vi "AxisControl.vi"(0 "String in":string, 1 "AxisBounds":T5={"Min"={"Auto"=TRUE, "Value"=0.0}, "Max"={"Auto"=TRUE, "Value"=0.0}}, 2 "Time Format String":string, 3 "ticsAndGrids":T2={"tics"={"ticMin"=0.0, "ticStep"=0.0, "ticMax"=0.0, "minorDivsPerMajor"=2, "ticSpacing"=enum."Auto Tics", "ticPosition"=enum."Inside, no mirror"}, "Grids"={"Gridlines"=enum."Major grid", "Zeroaxis"=enum."No zero axis"}, "Mapping"=enum."Lin"}, 5 "Axis":T7="x", 7 "Time format?":bool, 9 "ShowNumbers?":bool=TRUE, 11 "ShowLabel?":bool=TRUE, 12 "Axis Label":string, 13 "DataSpan":cluster{"Max":dbl, "Min":dbl}, 14 "AdditionalTics":dbl[](array[numeric])) -> (4 "String out":string, 6 "Commands":T1)   [LabVIEW 2015]
uses:
  axisName.ctl
  minAndMax.ctl
  AutoManualNumber.ctl
  ticsAndGrids.ctl
  tics.ctl
  grids.ctl
  commandArray.ctl
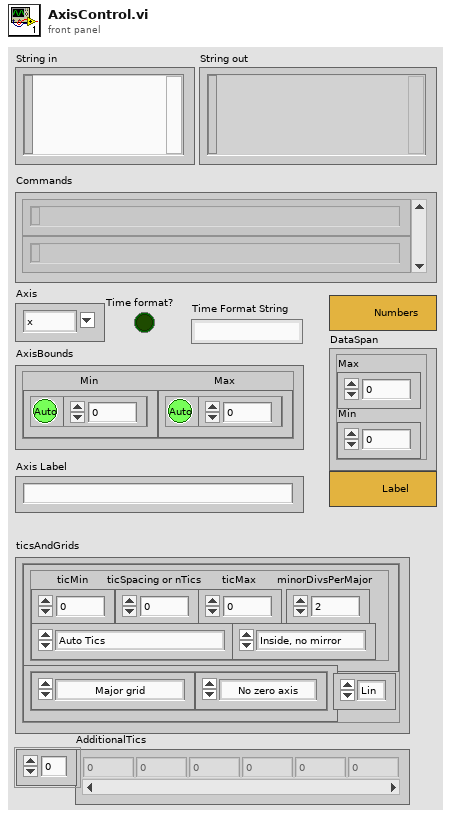
[diagram p1: front panel]
types:
  T1 = typedef "commandArray.ctl" = string[]
  T2 = typedef "ticsAndGrids.ctl" = cluster{"tics":T3, "Grids":T4, "Mapping":enum8{"Lin", "Log"}}
  T3 = typedef "tics.ctl" = cluster{"ticMin":dbl, "ticStep":dbl, "ticMax":dbl, "minorDivsPerMajor":i32, "ticSpacing":enum16{"Auto Tics", "Fixed spacing", "Fixed Minimum and Spacing", "Start, Spacing and Maximum", "Approx n Tics (rounded)"}, "ticPosition":enum16{"Inside, no mirror", "Inside, mirrored", "Outside, no mirror", "Outside, mirrored", "Invisible"}}
  T4 = typedef "grids.ctl" = cluster{"Gridlines":enum16{"No grids", "Major grid", "Minor grid", "Major and Minor"}, "Zeroaxis":enum16{"No zero axis", "Show zero axis"}}
  T5 = typedef "minAndMax.ctl" = cluster{"Min":T6, "Max":T6}
  T6 = typedef "AutoManualNumber.ctl" = cluster{"Auto":bool, "Value":dbl}
  T7 = typedef "axisName.ctl" = string
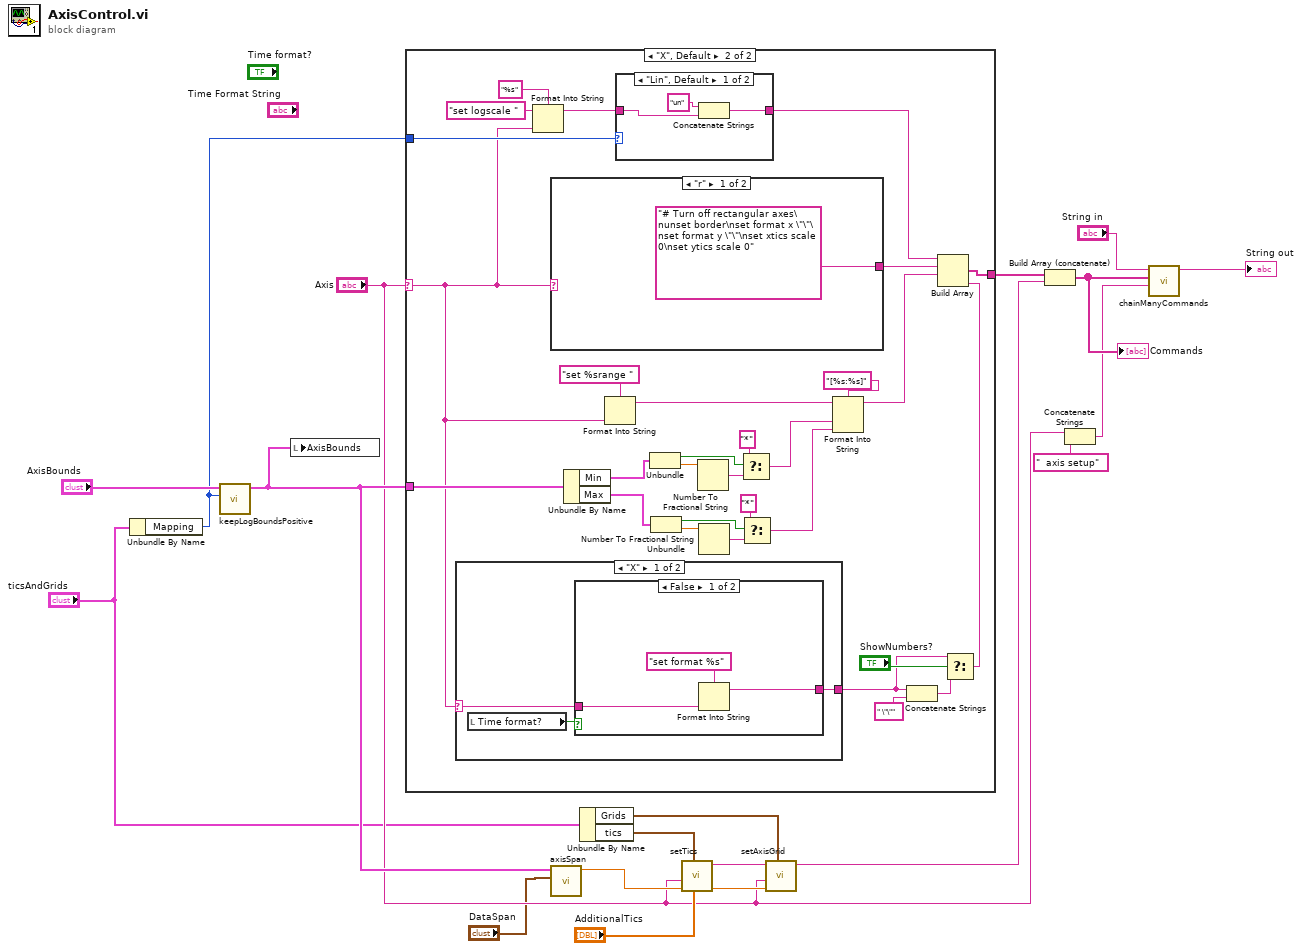
[diagram p0: block diagram]
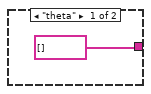
[diagram p2: hidden frame]
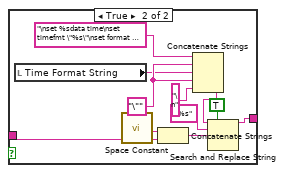
[diagram p3: hidden frame]
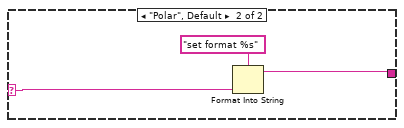
[diagram p4: hidden frame]
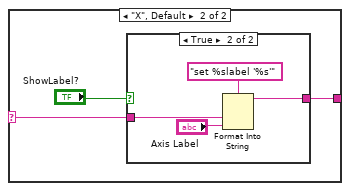
[diagram p6: hidden frame]
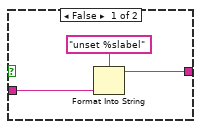
[diagram p7: hidden frame]
diagram:
  n1 = Unbundle By Name("ticsAndGrids") -> ("Mapping"=w3:enum8{"Lin", "Log"})
  n2 = call "keepLogBoundsPositive.vi"("Mapping"=w3, "AxisBounds in"="AxisBounds") -> ("AxisBounds out"=w8:T5)  [unwired: 9 in]
  n3 = local write "AxisBounds"(w8) -> ()
  n4 = case shown="\"X\", Default" "Axis" {
    selector: "Axis" -> [_ w22]
    tunnel: [string[] [] w44] -> w16
    tunnel: w8 -> [_ w28]
    tunnel: w3 -> [_ w27]
    frame "theta" {
    }
    frame "X", Default {
      n5 = case shown="\"X\"" w22 {
        selector: w22 -> [w51 w69]
        tunnel: [w52 w68] -> w21
        frame "X" {
          n6 = local read "Time format?"() -> (w53:bool)
          n7 = case shown="False" w53 {
            tunnel: [w55 w63] -> w52
            tunnel: w51 -> [w54 w62]
            frame False {
              n8 = Format Into String(format string="set format %s", w54) -> (resulting string=w55:string)  [unwired: 2 in, 1 out]
            }
            frame True {
              w60 = "\""
              n9 = local read "Time Format String"() -> (w59:string)
              n10 = call <vilib>:"Space Constant.vi"() -> ("String"=w66:string)
              n11 = Concatenate Strings(w66, w62) -> (w67:string)
              n12 = Concatenate Strings("\nset %sdata time\nset timefmt \"%s\"\nset format %s ", w60, w59, w60, "\n" ("string")) -> (w57:string)
              n13 = Search and Replace String(replace all?=TRUE ("replace all? (F)"), input string=w57, search string=" %s", replace string=w67) -> (result string=w63:string)  [unwired: 4 in, 3 out]
            }
          }
        }
        frame "Polar", Default {
          n14 = Format Into String(format string="set format %s", w69) -> (resulting string=w68:string)  [unwired: 2 in, 1 out]
        }
      }
      n15 = Format Into String(format string="%s", initial string="set logscale ", w22) -> (resulting string=w24:string)  [unwired: 1 in, 1 out]
      n16 = case shown="\"r\"" w22 {
        selector: w22 -> [_ w76]
        tunnel: ["# Turn off rectangular axes\nunset border\nset format x \"\"\nset format y \"\"\nset xtics scale 0\nset ytics scale 0" w77] -> w42
        frame "r" {
        }
        frame "X", Default {
          n17 = case shown="True" "ShowLabel?" {
            tunnel: w76 -> [w80 w83]
            tunnel: [w79 w82] -> w77
            frame False {
              n18 = Format Into String(format string="unset %slabel", w80) -> (resulting string=w79:string)  [unwired: 2 in, 1 out]
            }
            frame True {
              n19 = Format Into String(format string="set %slabel '%s'", w83, "Axis Label") -> (resulting string=w82:string)  [unwired: 2 in, 1 out]
            }
          }
        }
      }
      n20 = Unbundle By Name(w28) -> ("Min"=w30:T6, "Max"=w29:T6)
      n21 = Format Into String(format string="set %srange ", w22) -> (resulting string=w49:string)  [unwired: 2 in, 1 out]
      n22 = case shown="\"Lin\", Default" w27 {
        tunnel: [w72 w74] -> w23
        tunnel: w24 -> [w73 w74]
        frame "Lin", Default {
          n23 = Concatenate Strings("un" ("string"), w73) -> (w72:string)
        }
        frame "Log" {
        }
      }
      n24 = Unbundle(w30) -> ("Auto"=w37:bool, "Value"=w39:dbl)
      n25 = Unbundle(w29) -> ("Auto"=w35:bool, "Value"=w33:dbl)
      n26 = Number To Fractional String(number=w39) -> (F-format string=w40:string)  [unwired: 3 in]
      n27 = Number To Fractional String(number=w33) -> (F-format string=w32:string)  [unwired: 3 in]
      n28 = Select(t="*", s=w37, f=w40) -> (s? t:f=w36:string)
      n29 = Select(t="*", s=w35, f=w32) -> (s? t:f=w31:string)
      n30 = Format Into String(format string="[%s:%s]", initial string=w49, w36, w31) -> (resulting string=w48:string)  [unwired: 1 in, 1 out]
      n31 = Concatenate Strings(w21, " \"\"" ("format string")) -> (w45:string)
      n32 = Select(t=w21, s="ShowNumbers?", f=w45) -> (s? t:f=w43:string)
      n33 = Build Array(w23, w42, w48, w43) -> (w44:string[])
    }
  }
  n34 = call "axisSpan.vi"("DataSpan"="DataSpan", "AxisBounds"=w8) -> ("ActualSpan"=w10:dbl)  [unwired: 9 in]
  n35 = Unbundle By Name("ticsAndGrids") -> ("Grids"=w17:T4, "tics"=w18:T3)
  n36 = call "setTics.vi"("AdditionalTics"="AdditionalTics", "tics"=w18, "AxisSpan"=w10, "Axis"="Axis") -> ("polarGrid"=w14:dbl, "String out"=w19:string)  [unwired: 6 in]
  n37 = call "setAxisGrid.vi"("Grids"=w17, "polarGridAngle"=w14, "Axis"="Axis", "String in"=w19) -> ("String out"=w15:string)  [unwired: 7 in]
  n38 = Build Array (concatenate)(w16, w15) -> (w11:string[])
  "Commands" <- w11
  n39 = Concatenate Strings("Axis", "  axis setup" ("string")) -> (w6:string)
  n40 = call "chainManyCommands.vi"("Comments"=w6, "CommandArray"=w11, "String in in"="String in") -> ("String out"=→"String out":string)  [unwired: 8 in]
